vi "Zstack Save Image.vi"(8 "error in (no error)":errorcluster, 9 "Dataset base-path":path, 10 "Imaging Protocol":T1, 11 "Image Array":T2) -> (0 "error out":errorcluster)   [LabVIEW 2017]
uses:
  User Interface/Queue/Live graphs queue/Typedefs/Live imaging queue element.ctl
  <vilib>/vision/Image Controls.llb/IMAQ Image.ctl
  Typedefs/Imaging Protocols enum.ctl
  <vilib>/vision/NI_Vision_Development_Module.lvlib
panel:
  out "Array":path[](array[path])
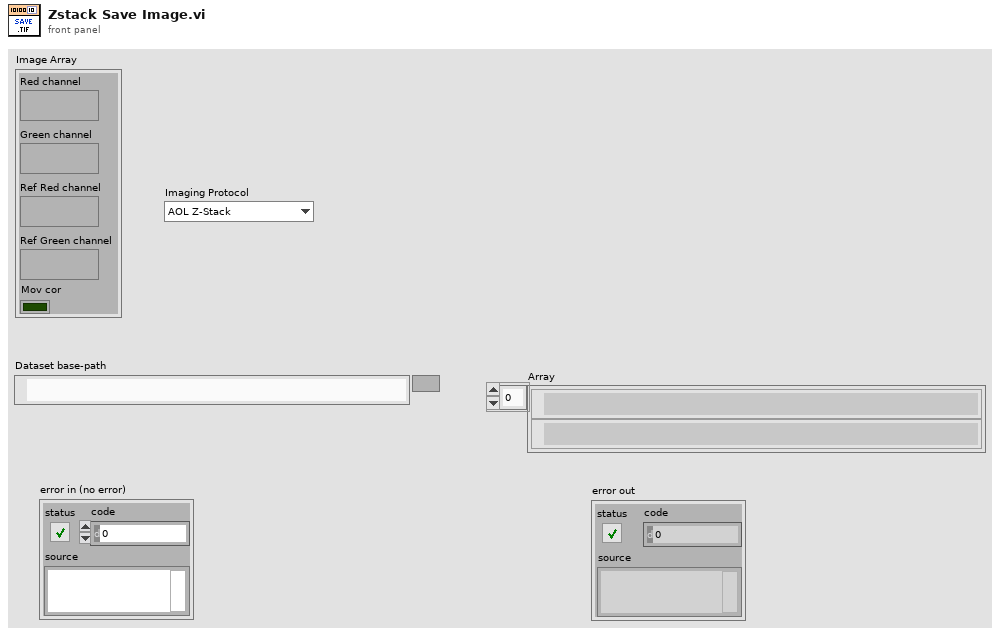
[diagram p1: front panel]
types:
  T1 = typedef "Imaging Protocols enum.ctl" = enum16{"AOL Z-Stack", "Motor Z Stack", "Parameter Sweep", "Functional Acquisition", "Single Plane Acquisition", "Volume Acquisition", "Live Imaging", "Live Plane Imaging", "Live Volume Imaging"}
  T2 = typedef "Live imaging queue element.ctl" = cluster{"Red channel":T3, "Green channel":T3, "Ref Red channel":T3, "Ref Green channel":T3, "Mov cor":bool}
  T3 = typedef "IMAQ Image.ctl" = refnum<image>
  T4 = typedef "Fixed strings.ctl" = cluster{"ROI file name":string, "Normalised ROI file name":string, "Zplane Pockels values file name":string, "Functional data folder name":string, "Experiment Header file name":string, "Z-stack images folder name":string, "Groups setup rel. path":string, "Groups text file rel. path":string, "TDMS files folder name (F.img)":string, "TDMS files folder name (V.acq)":string, "TDMS files folder name (Pl.acq)":string, "Cycle rel times sequence file":string, "Dynamically called VIs folder name":string, "Time Series folder base name":string, "Parameter Sweep":string}
  T5 = cluster{"Rows Per Strip":i32, "Photometric":i32, "Compression Type":i32}
  T6 = typedef "Image Type" = u32
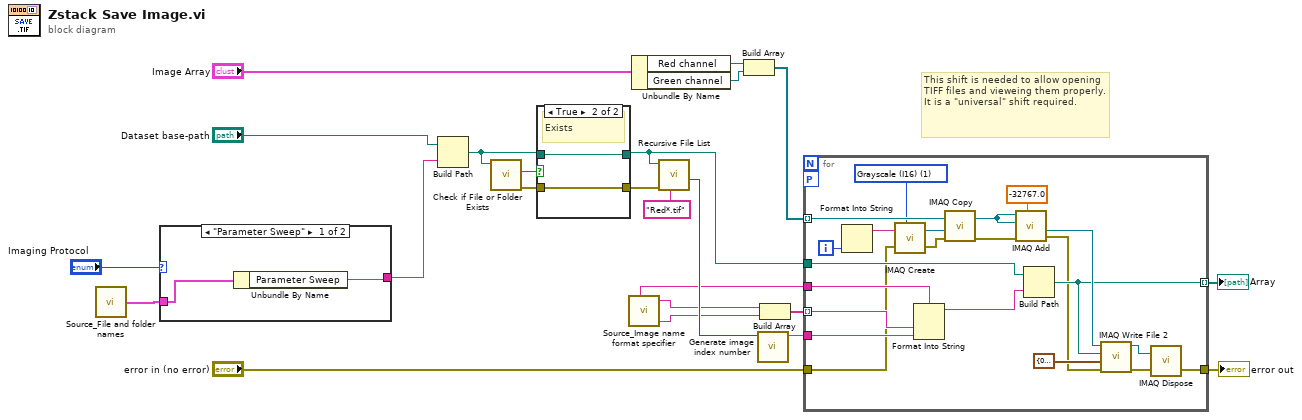
[diagram p0: block diagram]
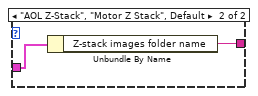
[diagram p2: hidden frame]
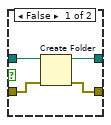
[diagram p3: hidden frame]
diagram:
  # "This shift is needed to allow opening TIFF files and vieweing them properly.\nIt is a \"universal\" shift required."
  n1 = call "Source_File and folder names.vi"() -> ("Fixed strings"=w1:T4)  [unwired: 1 in]
  n2 = case shown="\"Parameter Sweep\"" "Imaging Protocol" {
    tunnel: [w24 w27] -> w9
    tunnel: w1 -> [w25 w26]
    frame "Parameter Sweep" {
      n3 = Unbundle By Name(w25) -> ("Parameter Sweep"=w24:string)
    }
    frame "AOL Z-Stack", "Motor Z Stack", Default {
      n4 = Unbundle By Name(w26) -> ("Z-stack images folder name"=w27:string)
    }
  }
  n5 = Build Path(base path="Dataset base-path", name or relative path=w9) -> (appended path=w18:path)
  n6 = call <vilib>:"Check if File or Folder Exists.vi"("path"=w18) -> ("error out"=w16:errorcluster, "file or folder exists?"=w17:bool)  [unwired: 8 in, 1 out]
  n7 = case shown="True" w17 {
    tunnel: [w31 w32] -> w19
    tunnel: w18 -> [w30 w32]
    tunnel: w16 -> [w29 w33]
    tunnel: [w28 w33] -> w15
    frame False {
      n8 = Create Folder(path (use dialog)=w30, error in=w29) -> (created path=w31:path, error out=w28:errorcluster)  [unwired: 1 in, 1 out]
    }
    frame True {
      # "Exists"
    }
  }
  n9 = call "Source_Image name format specifier.vi"() -> ("Z-Stack Image name format specifier"=w11:string, "Red channel name"=w8:string, "Green channel name"=w7:string)  [unwired: 5 in]
  n10 = Unbundle By Name("Image Array") -> ("Red channel"=w4:T3, "Green channel"=w5:T3)
  n11 = call <vilib>:"Recursive File List.vi"("pattern"="Red*.tif", "error in (no error)"=w15, "Folder Path"=w19) -> ("Number of Files"=w14:i32)  [unwired: 4 in, 4 out]
  n12 = Build Array(w4, w5) -> (w3:T3[])
  n13 = call "Generate image index number.vi"("FOR loop iteration or existing number of files"=w14) -> ("Number in string representation (padded with zeroes)"=w13:string)  [unwired: 10 in]
  n14 = Build Array(w8, w7) -> (w10:string[])
  n15 = for {
    tunnel: w19 -> [w55]
    tunnel: w10 -> [w53] mode=indexing
    workers-P: _ -> [_]
    tunnel: "error in (no error)" -> [w42]
    tunnel: [w38] -> w21
    tunnel: w13 -> [w52]
    tunnel: [w50] -> w12 mode=indexing
    tunnel: w11 -> [w49]
    tunnel: w3 -> [w40] mode=indexing
    i -> [w35]
    w34 = T6 1 items=["Grayscale (U8)", "Grayscale (I16)", "Grayscale (SGL)", "Complex (CSG)", "RGB (U32)", "HSL (U32)", "RGB (U64)", "Grayscale (U16)"] ("Image Type")
    n16 = Format Into String(w35) -> (resulting string=w36:string)  [unwired: 3 in, 1 out]
    n17 = call "IMAQ Create"("Image Name"=w36, "Image Type"=w34, "error in (no error)"=w42) -> ("New Image"=w46:T3, "error out"=w44:errorcluster)  [unwired: 2 in]
    n18 = Format Into String(format string=w49, w53, w52) -> (resulting string=w51:string)  [unwired: 2 in, 1 out]
    n19 = call "IMAQ Copy"("error in (no error)"=w44, "Image Dst"=w46, "Image Src"=w40) -> ("error out"=w43:errorcluster, "Image Dst Out"=w45:T3)  [unwired: 3 in]
    n20 = call "IMAQ Add"("Image Src A"=w45, "Constant"=-32767.0, "Image Dst"=w45, "error in (no error)"=w43) -> ("Image Dst Out"=w54:T3, "error out"=w41:errorcluster)  [unwired: 3 in]
    n21 = Build Path(base path=w55, name or relative path=w51) -> (appended path=w50:path)
    n22 = call-poly "IMAQ Write File 2"("error in (no error)"=w41, "TIFF Options"=T5 {"Rows Per Strip"=0, "Photometric"=1, "Compression Type"=0}, "File Path"=w50, "Image"=w54) -> ("error out"=w39:errorcluster, "Image Out (duplicate)"=w37:T3)  [unwired: 6 in]
    n23 = call "IMAQ Dispose"("Image"=w37, "error in (no error)"=w39) -> ("error out"=w38:errorcluster)  [unwired: 4 in]
  }
  "error out" <- w21
  "Array" <- w12
